vi "PH_Revolver-GUI_6P.ProcPeriodic.vi"(0 "i ref in":refnum<vi>, 3 "ms timeout (100)":i32=100, 5 "error in (no error)":errorcluster) -> (14 "i ref out":refnum<vi>, 17 "timed out":bool, 19 "error out":errorcluster)   [LabVIEW 2014, in "PH_Revolver-GUI_6P.lvlib"]
doc: "This method serves to periodically do things like reading values from the HW. Methods that should be executed periodically should be called from THIS methode. Add code here."
uses:
  PH_Revolver-GUI_6P.lvlib
  PH_Basics/PH_AxisGUI_BaseClass/PH_AxisGUI_BaseClass.lvlib
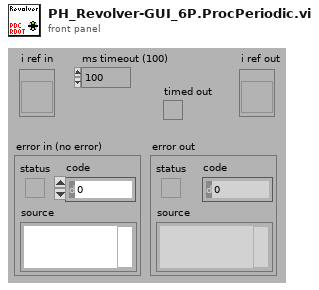
[diagram p1: front panel]
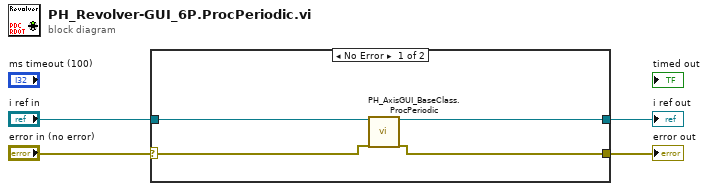
[diagram p0: block diagram]
diagram:
  n1 = case shown="No Error" "error in (no error)" {
    selector: "error in (no error)" -> [w6 w10]
    tunnel: [w5 w10] -> w3
    tunnel: [w7 w9] -> w2
    tunnel: "i ref in" -> [w8 w9]
    frame No Error {
      n2 = call "PH_AxisGUI_BaseClass.ProcPeriodic.vi"("i ref in"=w8, "error in (no error)"=w6) -> ("i ref out"=w7:refnum<vi>, "error out"=w5:errorcluster)  [unwired: 15 in, 1 out]
    }
    frame Error {
    }
  }
  "error out" <- w3
  "i ref out" <- w2
